vi "WKLXF25 St 60 PLC Data 2.0.vi"(9 "PLC string read Tags":T1={"Serial Number"={"Tag Name"="S060.PXI.Signals.PlltData.SN", "Network Path"="172.15.51.1,1,0", "use opc"=FALSE, "DataSocket Reference"={"CWDSLib._DCWDataSocket"=refnum, "CWDSLib._DCWData"=refnum, "OnDataUpdated"=0, "OnStatusUpdated"=0}}, "Pallet Number"={"Tag Name"="S060.PXI.Signals.PlltData.SN", "Network Path"="172.15.51.1,1,0", "use opc"=FALSE, "DataSocket Reference"={"CWDSLib._DCWDataSocket"=refnum, "CWDSLib._DCWData"=refnum, "OnDataUpdated"=0, "OnStatusUpdated"=0}}, "Inalfa Part Number"={"Tag Name"="S060.PXI.Signals.PlltData.SN", "Network Path"="172.15.51.1,1,0", "use opc"=FALSE, "DataSocket Reference"={"CWDSLib._DCWDataSocket"=refnum, "CWDSLib._DCWData"=refnum, "OnDataUpdated"=0, "OnStatusUpdated"=0}}, "Shade Color"={"Tag Name"="S060.PXI.Signals.PlltData.SN", "Network Path"="172.15.51.1,1,0", "use opc"=FALSE, "DataSocket Reference"={"CWDSLib._DCWDataSocket"=refnum, "CWDSLib._DCWData"=refnum, "OnDataUpdated"=0, "OnStatusUpdated"=0}}, "Model Type"={"Tag Name"="S060.PXI.Signals.PlltData.SN", "Network Path"="172.15.51.1,1,0", "use opc"=FALSE, "DataSocket Reference"={"CWDSLib._DCWDataSocket"=refnum, "CWDSLib._DCWData"=refnum, "OnDataUpdated"=0, "OnStatusUpdated"=0}}, "Customer Number"={"Tag Name"="S060.PXI.Signals.PlltData.SN", "Network Path"="172.15.51.1,1,0", "use opc"=FALSE, "DataSocket Reference"={"CWDSLib._DCWDataSocket"=refnum, "CWDSLib._DCWData"=refnum, "OnDataUpdated"=0, "OnStatusUpdated"=0}}, "Part History Number"={"Tag Name"="S060.PXI.Signals.PlltData.SN", "Network Path"="172.15.51.1,1,0", "use opc"=FALSE, "DataSocket Reference"={"CWDSLib._DCWDataSocket"=refnum, "CWDSLib._DCWData"=refnum, "OnDataUpdated"=0, "OnStatusUpdated"=0}}, "Shade 1 Barcode"={"Tag Name"="S060.PXI.Signals.PlltData.SN", "Network Path"="172.15.51.1,1,0", "use opc"=FALSE, "DataSocket Reference"={"CWDSLib._DCWDataSocket"=refnum, "CWDSLib._DCWData"=refnum, "OnDataUpdated"=0, "OnStatusUpdated"=0}}, "Shade 2 Barcode"={"Tag Name"="S060.PXI.Signals.PlltData.SN", "Network Path"="172.15.51.1,1,0", "use opc"=FALSE, "DataSocket Reference"={"CWDSLib._DCWDataSocket"=refnum, "CWDSLib._DCWData"=refnum, "OnDataUpdated"=0, "OnStatusUpdated"=0}}, "Manual Serial Number"={"Tag Name"="S060.PXI.Signals.PlltData.SN", "Network Path"="172.15.51.1,1,0", "use opc"=FALSE, "DataSocket Reference"={"CWDSLib._DCWDataSocket"=refnum, "CWDSLib._DCWData"=refnum, "OnDataUpdated"=0, "OnStatusUpdated"=0}}, "Manual Inalfa Part Number"={"Tag Name"="S060.PXI.Signals.PlltData.SN", "Network Path"="172.15.51.1,1,0", "use opc"=FALSE, "DataSocket Reference"={"CWDSLib._DCWDataSocket"=refnum, "CWDSLib._DCWData"=refnum, "OnDataUpdated"=0, "OnStatusUpdated"=0}}, "Manual Shade Color"={"Tag Name"="S060.PXI.Signals.PlltData.SN", "Network Path"="172.15.51.1,1,0", "use opc"=FALSE, "DataSocket Reference"={"CWDSLib._DCWDataSocket"=refnum, "CWDSLib._DCWData"=refnum, "OnDataUpdated"=0, "OnStatusUpdated"=0}}, "Manual Model Type"={"Tag Name"="S060.PXI.Signals.PlltData.SN", "Network Path"="172.15.51.1,1,0", "use opc"=FALSE, "DataSocket Reference"={"CWDSLib._DCWDataSocket"=refnum, "CWDSLib._DCWData"=refnum, "OnDataUpdated"=0, "OnStatusUpdated"=0}}, "Manual Customer Number"={"Tag Name"="S060.PXI.Signals.PlltData.SN", "Network Path"="172.15.51.1,1,0", "use opc"=FALSE, "DataSocket Reference"={"CWDSLib._DCWDataSocket"=refnum, "CWDSLib._DCWData"=refnum, "OnDataUpdated"=0, "OnStatusUpdated"=0}}, "Manual Part History Number"={"Tag Name"="S060.PXI.Signals.PlltData.SN", "Network Path"="172.15.51.1,1,0", "use opc"=FALSE, "DataSocket Reference"={"CWDSLib._DCWDataSocket"=refnum, "CWDSLib._DCWData"=refnum, "OnDataUpdated"=0, "OnStatusUpdated"=0}}, "iGPS SN 0"={"Tag Name"="S060.PXI.Signals.PlltData.SN", "Network Path"="172.15.51.1,1,0", "use opc"=FALSE, "DataSocket Reference"={"CWDSLib._DCWDataSocket"=refnum, "CWDSLib._DCWData"=refnum, "OnDataUpdated"=0, "OnStatusUpdated"=0}}, "iGPS SN 1"={"Tag Name"="S060.PXI.Signals.PlltData.SN", "Network Path"="172.15.51.1,1,0", "use opc"=FALSE, "DataSocket Reference"={"CWDSLib._DCWDataSocket"=refnum, "CWDSLib._DCWData"=refnum, "OnDataUpdated"=0, "OnStatusUpdated"=0}}, "iGPS SN 2"={"Tag Name"="S060.PXI.Signals.PlltData.SN", "Network Path"="172.15.51.1,1,0", "use opc"=FALSE, "DataSocket Reference"={"CWDSLib._DCWDataSocket"=refnum, "CWDSLib._DCWData"=refnum, "OnDataUpdated"=0, "OnStatusUpdated"=0}}, "iGPS SN 3"={"Tag Name"="S060.PXI.Signals.PlltData.SN", "Network Path"="172.15.51.1,1,0", "use opc"=FALSE, "DataSocket Reference"={"CWDSLib._DCWDataSocket"=refnum, "CWDSLib._DCWData"=refnum, "OnDataUpdated"=0, "OnStatusUpdated"=0}}, "iGPS SN 4"={"Tag Name"="S060.PXI.Signals.PlltData.SN", "Network Path"="172.15.51.1,1,0", "use opc"=FALSE, "DataSocket Reference"={"CWDSLib._DCWDataSocket"=refnum, "CWDSLib._DCWData"=refnum, "OnDataUpdated"=0, "OnStatusUpdated"=0}}, "iGPS SN 5"={"Tag Name"="S060.PXI.Signals.PlltData.SN", "Network Path"="172.15.51.1,1,0", "use opc"=FALSE, "DataSocket Reference"={"CWDSLib._DCWDataSocket"=refnum, "CWDSLib._DCWData"=refnum, "OnDataUpdated"=0, "OnStatusUpdated"=0}}, "iGPS SN 6"={"Tag Name"="S060.PXI.Signals.PlltData.SN", "Network Path"="172.15.51.1,1,0", "use opc"=FALSE, "DataSocket Reference"={"CWDSLib._DCWDataSocket"=refnum, "CWDSLib._DCWData"=refnum, "OnDataUpdated"=0, "OnStatusUpdated"=0}}, "iGPS SN 7"={"Tag Name"="S060.PXI.Signals.PlltData.SN", "Network Path"="172.15.51.1,1,0", "use opc"=FALSE, "DataSocket Reference"={"CWDSLib._DCWDataSocket"=refnum, "CWDSLib._DCWData"=refnum, "OnDataUpdated"=0, "OnStatusUpdated"=0}}, "iGPS SN 8"={"Tag Name"="S060.PXI.Signals.PlltData.SN", "Network Path"="172.15.51.1,1,0", "use opc"=FALSE, "DataSocket Reference"={"CWDSLib._DCWDataSocket"=refnum, "CWDSLib._DCWData"=refnum, "OnDataUpdated"=0, "OnStatusUpdated"=0}}, "iGPS SN 9"={"Tag Name"="S060.PXI.Signals.PlltData.SN", "Network Path"="172.15.51.1,1,0", "use opc"=FALSE, "DataSocket Reference"={"CWDSLib._DCWDataSocket"=refnum, "CWDSLib._DCWData"=refnum, "OnDataUpdated"=0, "OnStatusUpdated"=0}}} {"iGPS SN 9"."DataSocket Reference"."OnStatusUpdated" format="%.0x"; "iGPS SN 9"."DataSocket Reference"."OnDataUpdated" format="%.0x"; "iGPS SN 8"."DataSocket Reference"."OnStatusUpdated" format="%.0x"; "iGPS SN 8"."DataSocket Reference"."OnDataUpdated" format="%.0x"; "iGPS SN 7"."DataSocket Reference"."OnStatusUpdated" format="%.0x"; "iGPS SN 7"."DataSocket Reference"."OnDataUpdated" format="%.0x"; "iGPS SN 6"."DataSocket Reference"."OnStatusUpdated" format="%.0x"; "iGPS SN 6"."DataSocket Reference"."OnDataUpdated" format="%.0x"; "iGPS SN 5"."DataSocket Reference"."OnStatusUpdated" format="%.0x"; "iGPS SN 5"."DataSocket Reference"."OnDataUpdated" format="%.0x"; "iGPS SN 4"."DataSocket Reference"."OnStatusUpdated" format="%.0x"; "iGPS SN 4"."DataSocket Reference"."OnDataUpdated" format="%.0x"; "iGPS SN 3"."DataSocket Reference"."OnStatusUpdated" format="%.0x"; "iGPS SN 3"."DataSocket Reference"."OnDataUpdated" format="%.0x"; "iGPS SN 2"."DataSocket Reference"."OnStatusUpdated" format="%.0x"; "iGPS SN 2"."DataSocket Reference"."OnDataUpdated" format="%.0x"; "iGPS SN 1"."DataSocket Reference"."OnStatusUpdated" format="%.0x"; "iGPS SN 1"."DataSocket Reference"."OnDataUpdated" format="%.0x"; "iGPS SN 0"."DataSocket Reference"."OnStatusUpdated" format="%.0x"; "iGPS SN 0"."DataSocket Reference"."OnDataUpdated" format="%.0x"; "Manual Part History Number"."DataSocket Reference"."OnStatusUpdated" format="%.0x"; "Manual Part History Number"."DataSocket Reference"."OnDataUpdated" format="%.0x"; "Manual Customer Number"."DataSocket Reference"."OnStatusUpdated" format="%.0x"; "Manual Customer Number"."DataSocket Reference"."OnDataUpdated" format="%.0x"; "Manual Model Type"."DataSocket Reference"."OnStatusUpdated" format="%.0x"; "Manual Model Type"."DataSocket Reference"."OnDataUpdated" format="%.0x"; "Manual Shade Color"."DataSocket Reference"."OnStatusUpdated" format="%.0x"; "Manual Shade Color"."DataSocket Reference"."OnDataUpdated" format="%.0x"; "Manual Inalfa Part Number"."DataSocket Reference"."OnStatusUpdated" format="%.0x"; "Manual Inalfa Part Number"."DataSocket Reference"."OnDataUpdated" format="%.0x"; "Manual Serial Number"."DataSocket Reference"."OnStatusUpdated" format="%.0x"; "Manual Serial Number"."DataSocket Reference"."OnDataUpdated" format="%.0x"; "Shade 2 Barcode"."DataSocket Reference"."OnStatusUpdated" format="%.0x"; "Shade 2 Barcode"."DataSocket Reference"."OnDataUpdated" format="%.0x"; "Shade 1 Barcode"."DataSocket Reference"."OnStatusUpdated" format="%.0x"; "Shade 1 Barcode"."DataSocket Reference"."OnDataUpdated" format="%.0x"; "Part History Number"."DataSocket Reference"."OnStatusUpdated" format="%.0x"; "Part History Number"."DataSocket Reference"."OnDataUpdated" format="%.0x"; "Customer Number"."DataSocket Reference"."OnStatusUpdated" format="%.0x"; "Customer Number"."DataSocket Reference"."OnDataUpdated" format="%.0x"; "Model Type"."DataSocket Reference"."OnStatusUpdated" format="%.0x"; "Model Type"."DataSocket Reference"."OnDataUpdated" format="%.0x"; "Shade Color"."DataSocket Reference"."OnStatusUpdated" format="%.0x"; "Shade Color"."DataSocket Reference"."OnDataUpdated" format="%.0x"; "Inalfa Part Number"."DataSocket Reference"."OnStatusUpdated" format="%.0x"; "Inalfa Part Number"."DataSocket Reference"."OnDataUpdated" format="%.0x"; "Pallet Number"."DataSocket Reference"."OnStatusUpdated" format="%.0x"; "Pallet Number"."DataSocket Reference"."OnDataUpdated" format="%.0x"; "Serial Number"."DataSocket Reference"."OnStatusUpdated" format="%.0x"; "Serial Number"."DataSocket Reference"."OnDataUpdated" format="%.0x"}) -> (1 "No Data?":bool, 2 "Error String":string, 3 "PLC Data":T4)   [LabVIEW 2018]
uses:
  02.Type Def's/WKLXF25 St 60 PLC Data Control.ctl
  02.Type Def's/station plc read string tags.ctl
  05.UserVI's/type defs/plc path and tag.ctl
  <vilib>/Platform/dataskt.llb/DataSocket Reference Type.ctl
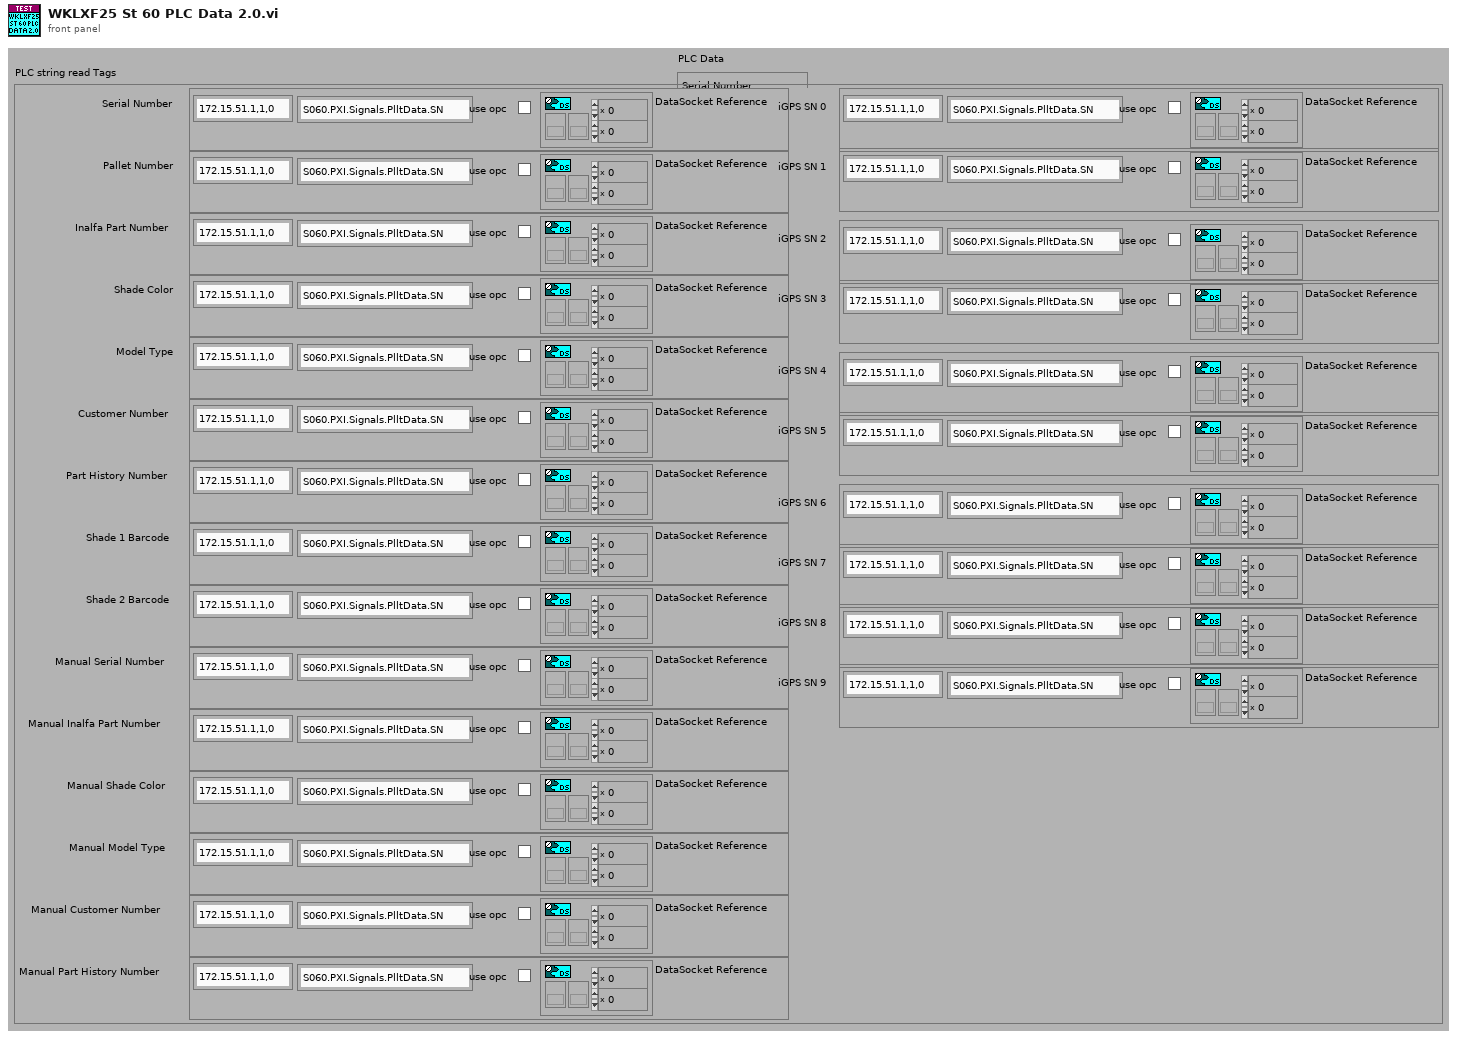
[diagram p1: front panel]
types:
  T1 = typedef "station plc read string tags.ctl" = cluster{"Serial Number":T2, "Pallet Number":T2, "Inalfa Part Number":T2, "Shade Color":T2, "Model Type":T2, "Customer Number":T2, "Part History Number":T2, "Shade 1 Barcode":T2, "Shade 2 Barcode":T2, "Manual Serial Number":T2, "Manual Inalfa Part Number":T2, "Manual Shade Color":T2, "Manual Model Type":T2, "Manual Customer Number":T2, "Manual Part History Number":T2, "iGPS SN 0":T2, "iGPS SN 1":T2, "iGPS SN 2":T2, "iGPS SN 3":T2, "iGPS SN 4":T2, "iGPS SN 5":T2, "iGPS SN 6":T2, "iGPS SN 7":T2, "iGPS SN 8":T2, "iGPS SN 9":T2}
  T2 = typedef "plc path and tag.ctl" = cluster{"Tag Name":string, "Network Path":string, "use opc":bool, "DataSocket Reference":T3}
  T3 = typedef "DataSocket Reference Type.ctl" = cluster{"CWDSLib._DCWDataSocket":refnum<k7>, "CWDSLib._DCWData":refnum<k7>, "OnDataUpdated":u32, "OnStatusUpdated":u32}
  T4 = typedef "WKLXF25 St 60 PLC Data Control.ctl" = cluster{"Serial Number":string, "Inalfa Part Number":string, "Sunshade Color":string, "Shade 1 Barcode":string, "Shade 2 Barcode":string, "Model Type":string, "Part History Number":string, "Customer Number":string}
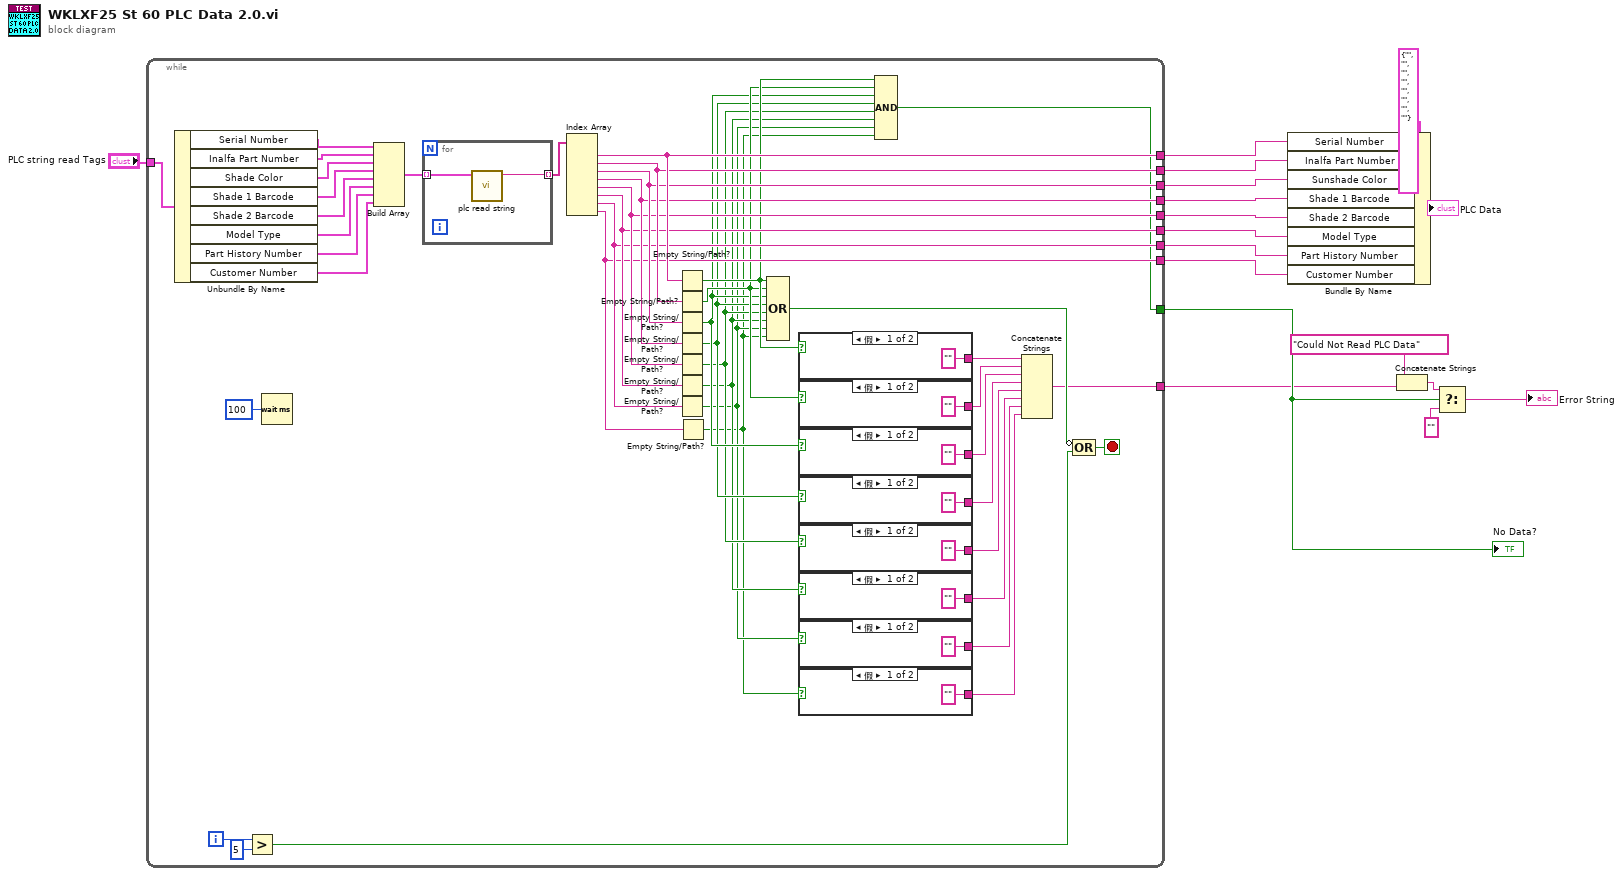
[diagram p0: block diagram]
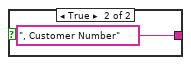
[diagram p2: hidden frame]
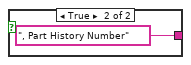
[diagram p3: hidden frame]
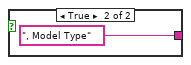
[diagram p4: hidden frame]
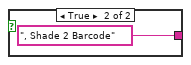
[diagram p5: hidden frame]
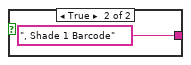
[diagram p6: hidden frame]
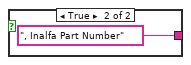
[diagram p7: hidden frame]
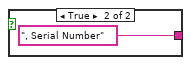
[diagram p8: hidden frame]
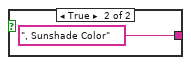
[diagram p9: hidden frame]
diagram:
  n1 = while {
    tunnel: [w18] -> w17
    tunnel: [w34] -> w12
    tunnel: [w33] -> w11
    tunnel: [w32] -> w10
    tunnel: [w31] -> w9
    tunnel: [w30] -> w8
    tunnel: [w29] -> w7
    tunnel: [w28] -> w6
    tunnel: [w27] -> w5
    tunnel: [w46] -> w2
    tunnel: "PLC string read Tags" -> [w45]
    i -> [w59]
    stop <- w56 stop-if-true
    n2 = Unbundle By Name(w45) -> ("Serial Number"=w44:T2, "Inalfa Part Number"=w43:T2, "Shade Color"=w42:T2, "Shade 1 Barcode"=w41:T2, "Shade 2 Barcode"=w40:T2, "Model Type"=w39:T2, "Part History Number"=w38:T2, "Customer Number"=w37:T2)
    n3 = Greater?(x=w59, y=5) -> (0:w57:bool)
    n4 = Wait (ms)(milliseconds to wait=u32 100) -> ()  [unwired: 1 out]
    n5 = Build Array(w44, w43, w42, w41, w40, w39, w38, w37) -> (w36:T2[])
    n6 = for {
      tunnel: w36 -> [w62] mode=indexing
      tunnel: [w61] -> w35 mode=indexing
      n7 = call "plc read string.vi"("addr,tag"=w62) -> ("Data"=w61:string)  [unwired: 9 in, 1 out]
    }
    n8 = Index Array(array=w35) -> (element #1=w34:string, element #2=w33:string, element #3=w32:string, element #4=w31:string, element #5=w30:string, element #6=w29:string, element #7=w28:string, element #8=w27:string)  [unwired: 8 in]
    n9 = Empty String/Path?(string/path=w34) -> (empty?=w26:bool)
    n10 = Empty String/Path?(string/path=w33) -> (empty?=w25:bool)
    n11 = Empty String/Path?(string/path=w32) -> (empty?=w24:bool)
    n12 = Empty String/Path?(string/path=w31) -> (empty?=w23:bool)
    n13 = Empty String/Path?(string/path=w30) -> (empty?=w22:bool)
    n14 = Empty String/Path?(string/path=w29) -> (empty?=w21:bool)
    n15 = Empty String/Path?(string/path=w28) -> (empty?=w20:bool)
    n16 = Empty String/Path?(string/path=w27) -> (empty?=w19:bool)
    n17 = Compound Arithmetic op=OR(w26, w25, w24, w23, w22, w21, w20, w19) -> (w55:bool)
    n18 = case shown="假" w26 {
      tunnel: ["" ", Serial Number"] -> w54
      frame False {
      }
      frame True {
      }
    }
    n19 = case shown="假" w25 {
      tunnel: ["" ", Inalfa Part Number"] -> w53
      frame False {
      }
      frame True {
      }
    }
    n20 = case shown="假" w24 {
      tunnel: ["" ", Sunshade Color"] -> w52
      frame False {
      }
      frame True {
      }
    }
    n21 = case shown="假" w23 {
      tunnel: ["" ", Shade 1 Barcode"] -> w51
      frame False {
      }
      frame True {
      }
    }
    n22 = case shown="假" w22 {
      tunnel: ["" ", Shade 2 Barcode"] -> w50
      frame False {
      }
      frame True {
      }
    }
    n23 = case shown="假" w21 {
      tunnel: ["" ", Model Type"] -> w49
      frame False {
      }
      frame True {
      }
    }
    n24 = case shown="假" w20 {
      tunnel: ["" ", Part History Number"] -> w48
      frame False {
      }
      frame True {
      }
    }
    n25 = case shown="假" w19 {
      tunnel: ["" ", Customer Number"] -> w47
      frame False {
      }
      frame True {
      }
    }
    n26 = Compound Arithmetic op=AND(w26, w25, w24, w23, w22, w21, w20, w19) -> (w18:bool)
    n27 = Concatenate Strings(w54, w53, w52, w51, w50, w49, w48, w47) -> (w46:string)
    n28 = Compound Arithmetic op=OR(invert w55, w57) -> (w56:bool)
  }
  "No Data?" <- w17
  n29 = Bundle By Name(cluster=T4 {"Serial Number"="", "Inalfa Part Number"="", "Sunshade Color"="", "Shade 1 Barcode"="", "Shade 2 Barcode"="", "Model Type"="", "Part History Number"="", "Customer Number"=""} ("St 60 PLC Data Control"), "Serial Number"=w12, "Inalfa Part Number"=w11, "Sunshade Color"=w10, "Shade 1 Barcode"=w9, "Shade 2 Barcode"=w8, "Model Type"=w7, "Part History Number"=w6, "Customer Number"=w5) -> (→"PLC Data":T4)
  n30 = Concatenate Strings("Could Not Read PLC Data" ("t"), w2) -> (w3:string)
  n31 = Select(t=w3, s=w17, f="") -> (s? t:f=→"Error String":string)
